vi "__Alicat SD_ManualSet_Individual.vi"(5 "USADO":bool[](array[boolean]), 6 "RANGOS":dbl[](array[numeric])=[0.0, 0.0, 0.0, 0.0, 0.0, 0.0, 0.0, 0.0] format="%.1g", 7 "Address (0.7)":i32, 8 "error in":errorcluster, 9 "SETPOINT":dbl format="%.1f", 10 "SETPOINT":dbl[](array[numeric])=[0.0, 0.0, 0.0, 0.0, 0.0, 0.0, 0.0, 0.0] format="%.1g", 11 "ID":string[](array[string])) -> (0 "error out":errorcluster, 2 "SETPOINT 2":dbl[](array[numeric]) format="%.1g")   [LabVIEW 2017]
uses:
  __Alicat SD_Hardware_Module.ctl
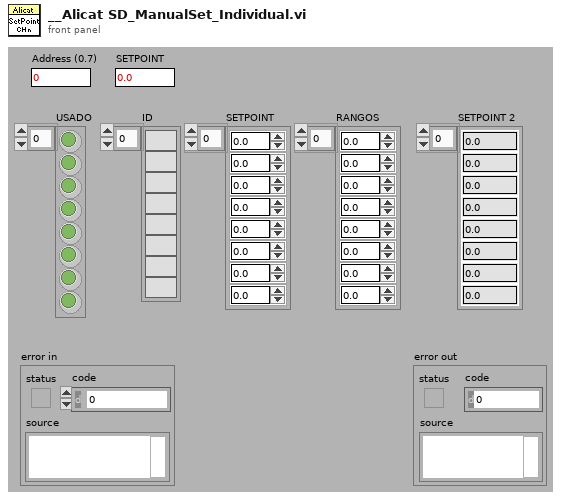
[diagram p1: front panel]
types:
  T1 = typedef "__Alicat SD_Hardware_Module.ctl" = enum16{"Initialize", "Send Setpoint", "Read Data", "Change Address", "Shutdown"}
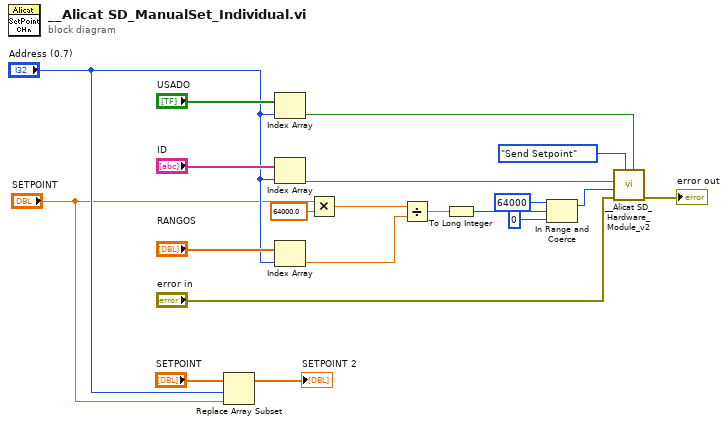
[diagram p0: block diagram]
diagram:
  n1 = Replace Array Subset(array="SETPOINT", new element="SETPOINT", index="Address (0.7)") -> (→"SETPOINT 2":dbl[])
  n2 = Index Array(array="USADO", index="Address (0.7)") -> (element=w1:bool)
  n3 = Index Array(array="ID", index="Address (0.7)") -> (element=w13:string)
  n4 = Index Array(array="RANGOS", index="Address (0.7)") -> (element=w11:dbl)
  n5 = Multiply(x="SETPOINT", y=64000.0) -> (x*y=w17:dbl)
  n6 = Divide(x=w17, y=w11) -> (x/y=w16:dbl)
  n7 = To Long Integer(number=w16) -> (32bit integer=w7:i32)
  n8 = In Range and Coerce(upper limit=64000 ("y"), x=w7, lower limit=0) -> (coerced(x)=w6:i32)  [unwired: 1 out]
  n9 = call "__Alicat SD_Hardware_Module_v2.vi"("Used ?"=w1, "Command"=__Alicat_SD_Hardware_Module."Send Setpoint", "error in (no error)"="error in", "SetPoint (64000=FullScale)"=w6, "Address"=w13) -> ("error out"=→"error out":errorcluster)  [unwired: 3 in, 3 out]
